vi "get_samples_vacak.vi"(0 "VISA Refnum in":refnum<visa-resource-name>, 1 "error in (no error)":errorcluster) -> (2 "VISA Refnum out":refnum<visa-resource-name>, 4 "error out":errorcluster)   [LabVIEW 2013]
uses:
  <vilib>/Analysis/NI_AALBase.lvlib
panel:
  in  "VISA Refnum in 3":refnum<visa-resource-name>
  in  "error in (no error) 3":errorcluster
  out "Waveform Graph 2":u8[][](graph)
  out "error out 2":errorcluster
  out "VISA Refnum out 2":refnum<visa-resource-name>
  in  "elemszam":u16
  in  "error in (no error) 2":errorcluster
  in  "VISA Refnum in 2":refnum<visa-resource-name>
  out "Waveform Graph":u8[][](graph)
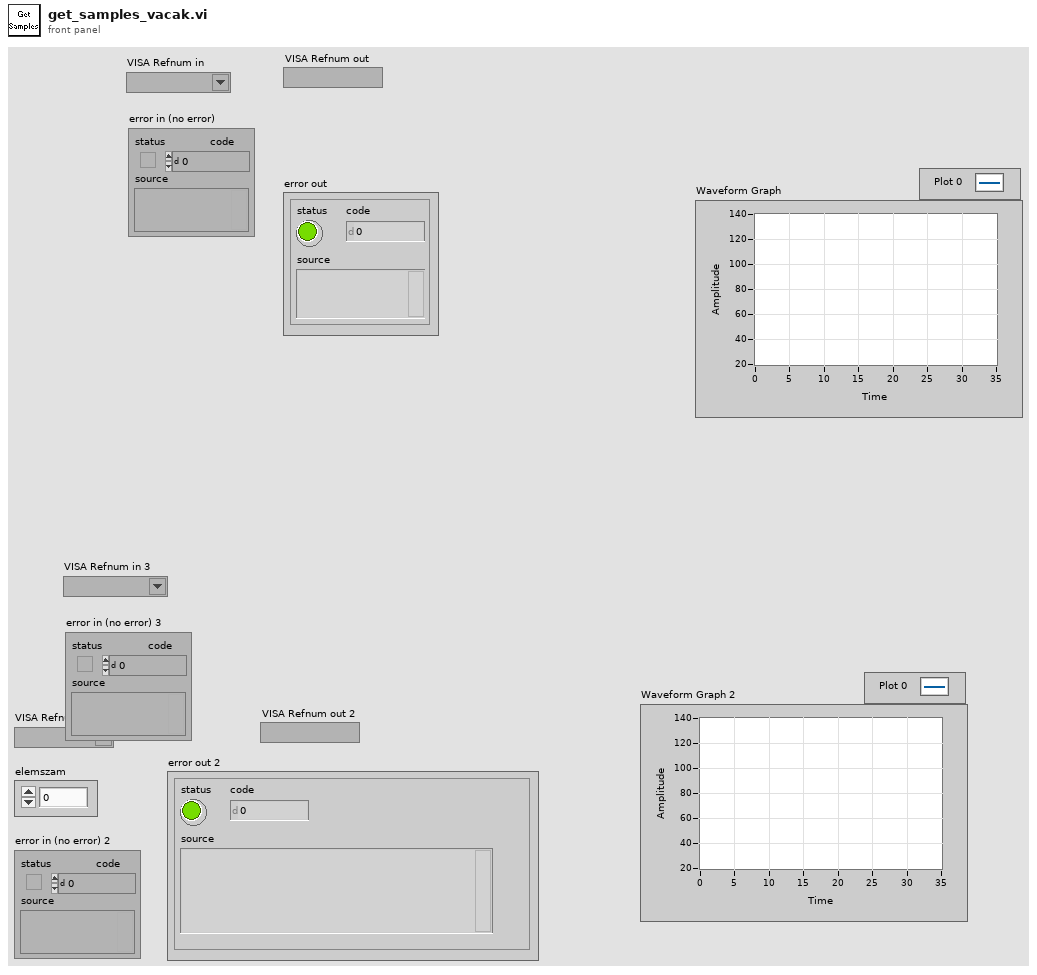
[diagram p1: front panel]
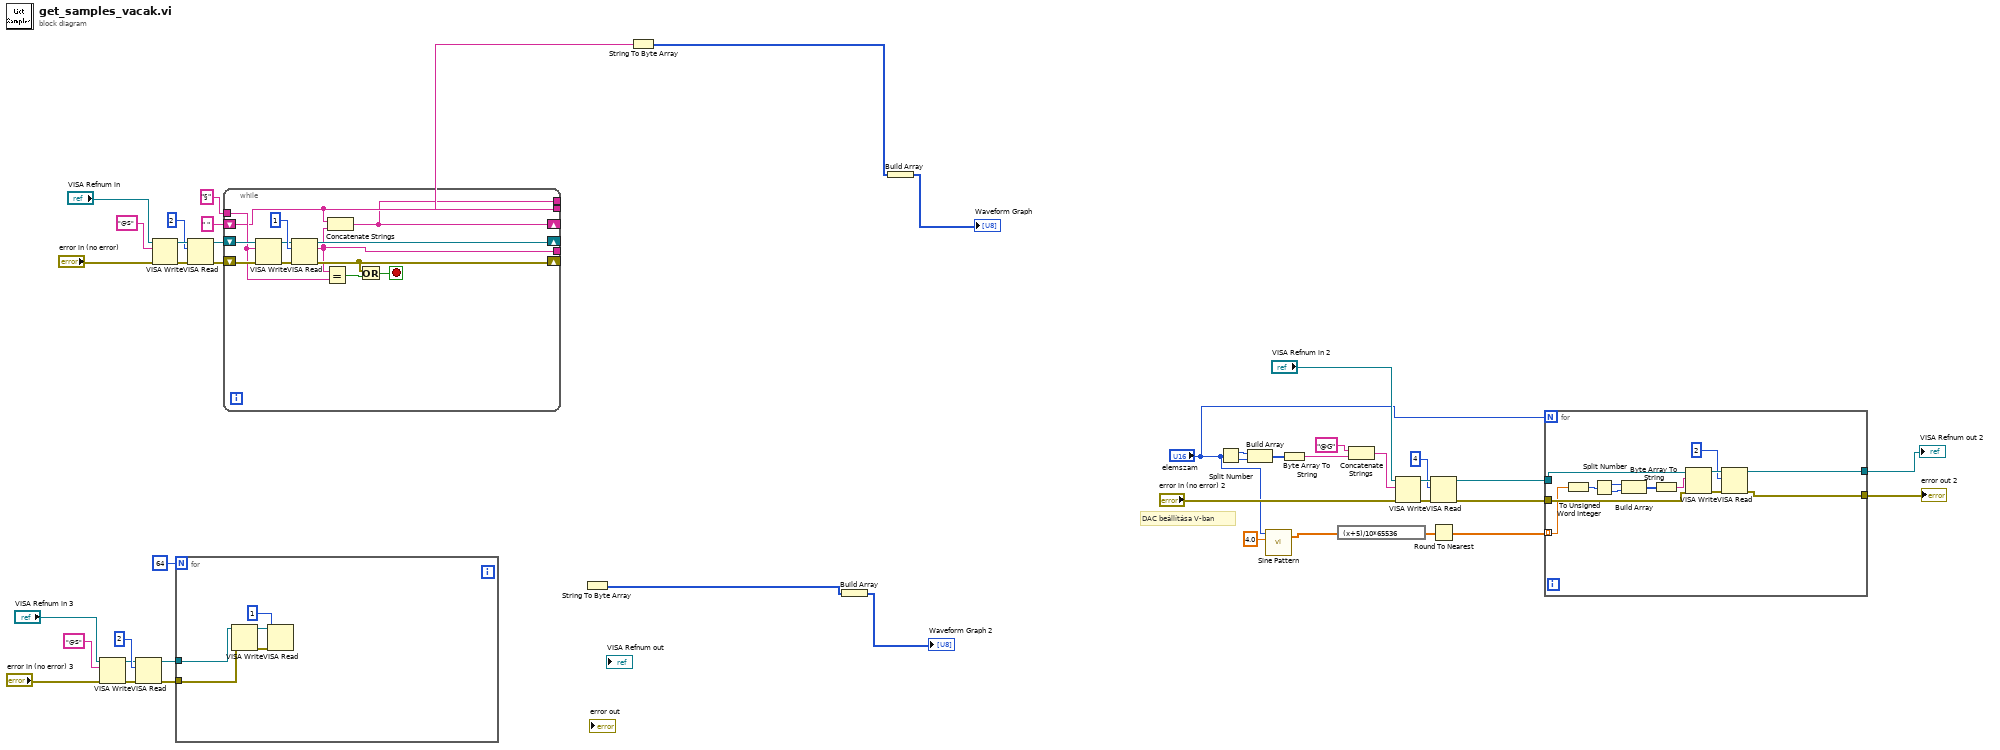
[diagram p0: block diagram]
diagram:
  # "DAC beállítása V-ban"
  n1 = VISA Write(VISA resource name="VISA Refnum in 3", write buffer="@S", error in (no error)="error in (no error) 3") -> (VISA resource name out=w6:refnum<visa-resource-name>, error out=w7:errorcluster)  [unwired: 1 out]
  n2 = VISA Read(VISA resource name=w6, byte count=u32 2, error in (no error)=w7) -> (VISA resource name out=w2:refnum<visa-resource-name>, error out=w1:errorcluster)  [unwired: 2 out]
  n3 = VISA Write(VISA resource name="VISA Refnum in", write buffer="@S", error in (no error)="error in (no error)") -> (VISA resource name out=w39:refnum<visa-resource-name>, error out=w38:errorcluster)  [unwired: 1 out]
  n4 = for {
    N: 64 -> [_]
    tunnel: w2 -> [w46]
    tunnel: w1 -> [w45]
    n5 = VISA Write(VISA resource name=w46, error in (no error)=w45) -> (VISA resource name out=w49:refnum<visa-resource-name>, error out=w48:errorcluster)  [unwired: 1 in, 1 out]
    n6 = VISA Read(VISA resource name=w49, byte count=u32 1, error in (no error)=w48) -> ()  [unwired: 4 out]
  }
  n7 = VISA Read(VISA resource name=w39, byte count=u32 2, error in (no error)=w38) -> (VISA resource name out=w37:refnum<visa-resource-name>, error out=w35:errorcluster)  [unwired: 2 out]
  n8 = while {
    tunnel: "§" ("write buffer") -> [w53]
    shift-right: [w59] -> _
    shift-left: w37 -> [w58]
    shift-right: [w55] -> _
    shift-left: w35 -> [w57]
    shift-right: [w51] -> _
    shift-left: " " ("string") -> [w52]
    tunnel: [w52] -> w34
    tunnel: [w51] -> _
    tunnel: [w50] -> _
    stop <- w56 stop-if-true
    n9 = VISA Write(VISA resource name=w58, write buffer=w53, error in (no error)=w57) -> (VISA resource name out=w61:refnum<visa-resource-name>, error out=w60:errorcluster)  [unwired: 1 out]
    n10 = VISA Read(VISA resource name=w61, byte count=u32 1, error in (no error)=w60) -> (VISA resource name out=w59:refnum<visa-resource-name>, read buffer=w50:string, error out=w55:errorcluster)  [unwired: 1 out]
    n11 = Equal?(x=w50, y=w53) -> (x = y?=w54:bool)
    n12 = Concatenate Strings(w52, w50) -> (w51:string)
    n13 = Or(x=w55, y=w54) -> (x .or. y?=w56:bool)
  }
  n14 = String To Byte Array() -> (unsigned byte array=w9:u8[])  [unwired: 1 in]
  n15 = String To Byte Array(string=w34) -> (unsigned byte array=w33:u8[])
  n16 = Build Array(w9) -> (→"Waveform Graph 2":u8[][])
  n17 = Build Array(w33) -> (→"Waveform Graph":u8[][])
  n18 = Split Number(x="elemszam") -> (hi(x)=w24:u8, lo(x)=w25:u8)
  n19 = Build Array(w24, w25) -> (w26:u8[])
  n20 = call <vilib>:"Sine Pattern.vi"("amplitude"=4.0, "samples"="elemszam") -> ("Sinusoidal Pattern"=w13:dbl[])  [unwired: 2 in, 1 out]
  n21 = Byte Array To String(unsigned byte array=w26) -> (string=w27:string)
  n22 = expression code="(x+5)/10*65536"(w13) -> (w16:dbl[])
  n23 = Concatenate Strings("@G" ("write buffer"), w27) -> (w20:string)
  n24 = VISA Write(VISA resource name="VISA Refnum in 2", write buffer=w20, error in (no error)="error in (no error) 2") -> (VISA resource name out=w22:refnum<visa-resource-name>, error out=w23:errorcluster)  [unwired: 1 out]
  n25 = VISA Read(VISA resource name=w22, byte count=u32 4, error in (no error)=w23) -> (VISA resource name out=w29:refnum<visa-resource-name>, error out=w28:errorcluster)  [unwired: 2 out]
  n26 = Round To Nearest(number=w16) -> (nearest integer value=w12:dbl[])
  n27 = for {
    N: "elemszam" -> [_]
    tunnel: w12 -> [w68] mode=indexing
    tunnel: w28 -> [w74]
    tunnel: w29 -> [w73]
    tunnel: [w64] -> w30
    tunnel: [w63] -> w31
    n28 = To Unsigned Word Integer(number=w68) -> (unsigned 16bit integer=w71:u16)
    n29 = Split Number(x=w71) -> (hi(x)=w69:u8, lo(x)=w70:u8)
    n30 = Build Array(w69, w70) -> (w72:u8[])
    n31 = Byte Array To String(unsigned byte array=w72) -> (string=w67:string)
    n32 = VISA Write(VISA resource name=w73, write buffer=w67, error in (no error)=w74) -> (VISA resource name out=w66:refnum<visa-resource-name>, error out=w75:errorcluster)  [unwired: 1 out]
    n33 = VISA Read(VISA resource name=w66, byte count=u32 2, error in (no error)=w75) -> (VISA resource name out=w64:refnum<visa-resource-name>, error out=w63:errorcluster)  [unwired: 2 out]
  }
  "VISA Refnum out 2" <- w30
  "error out 2" <- w31
